vi "INV A - Current Sense Test_v2.vi"(8 "error in (no error)":errorcluster, 11 "Control Board VISA":refnum<visa-resource-name>) -> (0 "error out":errorcluster, 3 "Sense UVW":dbl[](array[numeric]))   [LabVIEW 2022 SP3]
uses:
  Serial Board Com/Board Select.ctl
  Serial Board Com/ADCSelector BB.ctl
  Serial Board Com/ADCSelector GB.ctl
panel:
  in  "Board Select":T1
  out "Sense W":dbl
  out "Sense V":dbl
  out "Sense U":dbl
  out "INVA_ISENSE_W":bool
  out "INVA_ISENSE_V":bool
  out "INVA_ISENSE_U":bool
  in  "Message IN":string
  out "Message OUT":string
  out "VISA OUT":refnum<visa-resource-name>
  out "Result (color)":u32(colorbox)
  out "Result (bool)":bool
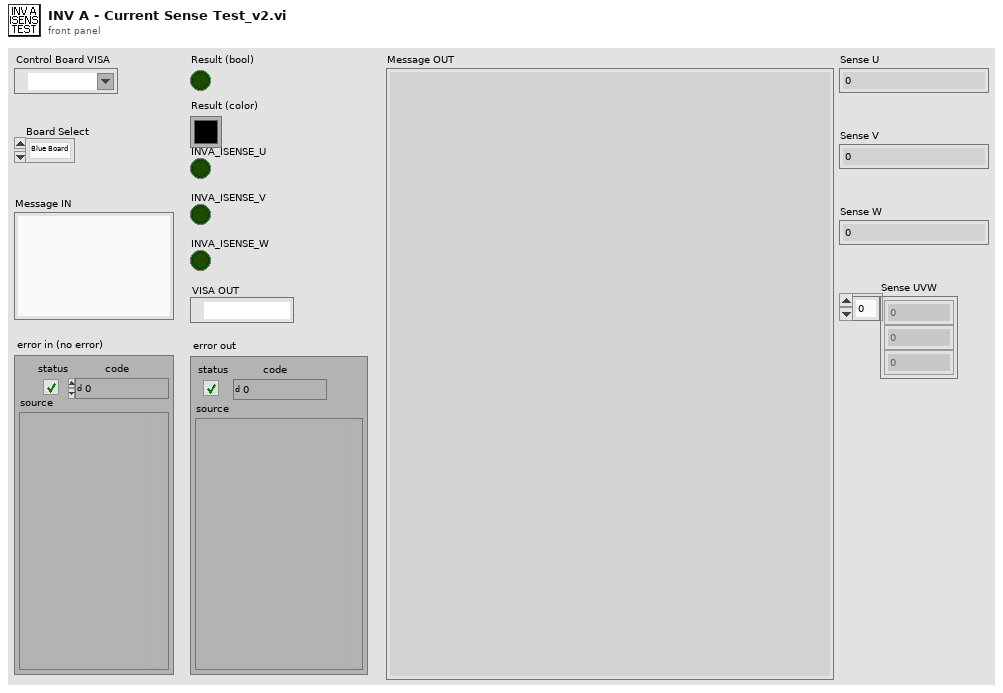
[diagram p1: front panel]
types:
  T1 = typedef "Board Select.ctl" = enum16{"Blue Board", "Green Board"}
  T2 = typedef "ADCSelector GB.ctl" = enum16{"INVA_ISENSE_U", "INVA_ISENSE_V", "INVA_ISENSE_W", "INVA_UDC", "INVA_TEMP", "HB_ISENSE", "AUX_ISENSE_U", "AUX_ISENSE_V", "AUX_ISENSE_W", "VLINE_AB", "VLINE_BC", "VLINE_CA", "REF_1P5V", "VSENSE_POS_24V", "VSENSE_POS_5V", "VSENSE_NEG_15V", "TEST_POINT", "INVB_ISENSE_U", "INVB_ISENSE_V", "INVB_ISENSE_W", "INVB_UDC", "INVB_TEMP", "HB_TEMP", "AUXA_TEMP", "AUXB_TEMP", "AUXC_TEMP", "VOUT_AB", "VOUT_BC", "VOUT_CA", "REF_2P5V", "VSENSE_POS_15V", "VSENSE_POS_3P3V", "NET_ANALYZER"}
  T3 = typedef "ADCSelector BB.ctl" = enum16{"INVA_ISENSE_U", "INVA_ISENSE_V", "INVA_ISENSE_W", "INVA_UDC", "INVA_TEMP", "HB_TEMP", "AUXB_TEMP", "VLINE_AB", "VLINE_BC", "VLINE_CA", "VSENSE_POS_24V", "VSENSE_POS_5V", "VSENSE_NEG_15V", "INVB_ISENSE_U", "INV_B_ISENSEV", "INVB_ISENSE_W", "INVB_UDC", "INVB_TEMP", "AUXA_TEMP", "AUXC_TEMP", "VOUT_AB", "VOUT_BC", "VOUT_CA", "VSENSE_POS_15V", "VSENSE_POS_3P3V", "TEST_POINT"}
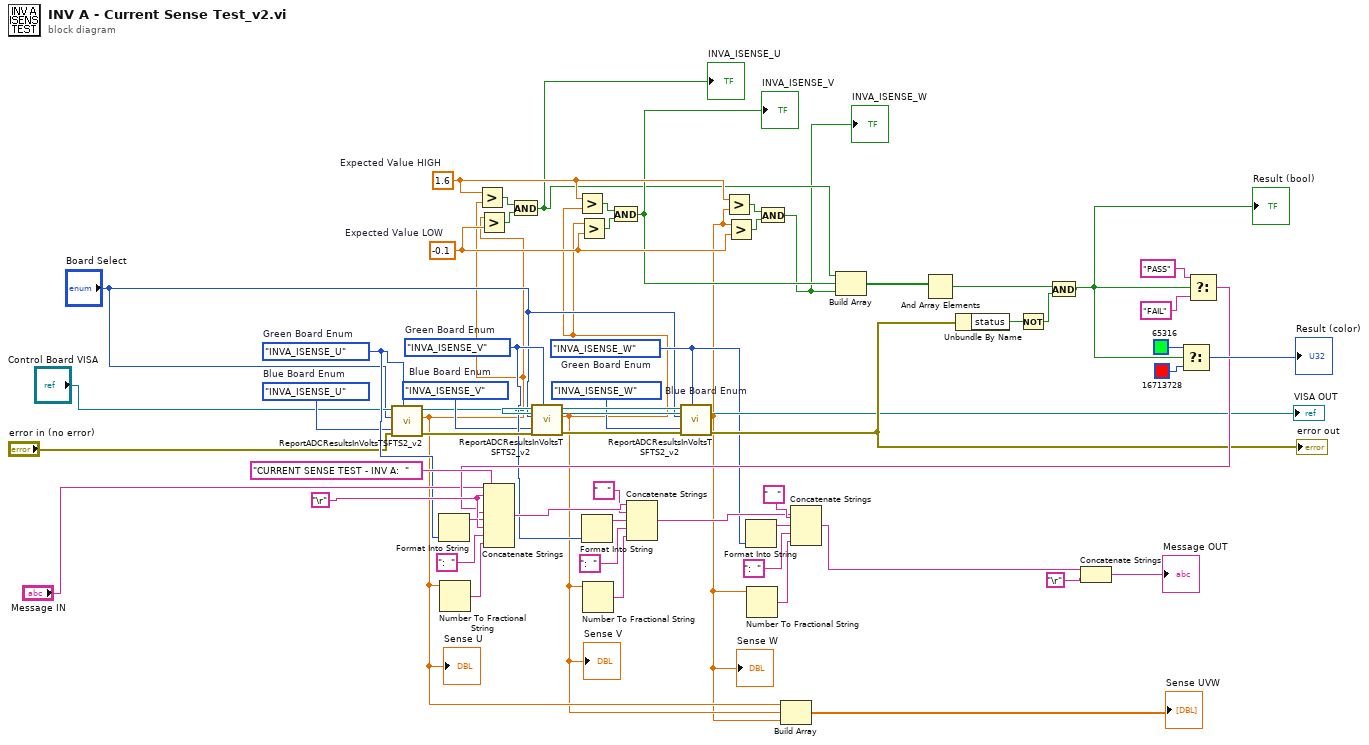
[diagram p0: block diagram]
diagram:
  w14 = ADCSelector_GB."INVA_ISENSE_W"  # Green Board Enum
  w15 = ADCSelector_GB."INVA_ISENSE_V"  # Green Board Enum
  w16 = ADCSelector_GB."INVA_ISENSE_U"  # Green Board Enum
  w21 = "\r"
  w36 = -0.1  # Expected Value LOW
  w35 = 1.6  # Expected Value HIGH
  w10 = ADCSelector_BB."INVA_ISENSE_W"  # Blue Board Enum
  w11 = ADCSelector_BB."INVA_ISENSE_V"  # Blue Board Enum
  w12 = ADCSelector_BB."INVA_ISENSE_U"  # Blue Board Enum
  n1 = call "ReportADCResultsInVoltsTSFTS2_v2.vi"("Blue Board Enum"=w12, "Green Board Enum"=w16, "error in (no error)"="error in (no error)", "Board Selector"="Board Select", "Control Board VISA"="Control Board VISA") -> ("error out"=w51:errorcluster, "Result"=w5:dbl, "Control Board VISA Out"=w7:refnum<visa-resource-name>)  [unwired: 3 in, 1 out]
  "Sense U" <- w5
  n2 = Format Into String(w16) -> (resulting string=w22:string)  [unwired: 3 in, 1 out]
  n3 = Number To Fractional String(number=w5) -> (F-format string=w24:string)  [unwired: 3 in]
  n4 = Greater?(x=w35, y=w5) -> (0:w42:bool)
  n5 = Greater?(x=w5, y=w36) -> (0:w41:bool)
  n6 = And(x=w42, y=w41) -> (x .and. y?=w33:bool)
  "INVA_ISENSE_U" <- w33
  n7 = call "ReportADCResultsInVoltsTSFTS2_v2.vi"("Blue Board Enum"=w11, "Green Board Enum"=w15, "error in (no error)"=w51, "Board Selector"="Board Select", "Control Board VISA"=w7) -> ("error out"=w50:errorcluster, "Result"=w4:dbl, "Control Board VISA Out"=w6:refnum<visa-resource-name>)  [unwired: 3 in, 1 out]
  "Sense V" <- w4
  n8 = Greater?(x=w35, y=w4) -> (0:w39:bool)
  n9 = Greater?(x=w4, y=w36) -> (0:w40:bool)
  n10 = Format Into String(w15) -> (resulting string=w47:string)  [unwired: 3 in, 1 out]
  n11 = Number To Fractional String(number=w4) -> (F-format string=w48:string)  [unwired: 3 in]
  n12 = And(x=w39, y=w40) -> (x .and. y?=w34:bool)
  "INVA_ISENSE_V" <- w34
  n13 = call "ReportADCResultsInVoltsTSFTS2_v2.vi"("Blue Board Enum"=w10, "Green Board Enum"=w14, "error in (no error)"=w50, "Board Selector"="Board Select", "Control Board VISA"=w6) -> ("error out"=w18:errorcluster, "Result"=w3:dbl, "Control Board VISA Out"=→"VISA OUT":refnum<visa-resource-name>)  [unwired: 3 in, 1 out]
  "error out" <- w18
  "Sense W" <- w3
  n14 = Greater?(x=w35, y=w3) -> (0:w38:bool)
  n15 = Greater?(x=w3, y=w36) -> (0:w37:bool)
  n16 = Format Into String(w14) -> (resulting string=w46:string)  [unwired: 3 in, 1 out]
  n17 = Number To Fractional String(number=w3) -> (F-format string=w45:string)  [unwired: 3 in]
  n18 = And(x=w38, y=w37) -> (x .and. y?=w32:bool)
  "INVA_ISENSE_W" <- w32
  n19 = Build Array(w5, w4, w3) -> (→"Sense UVW":dbl[])
  n20 = Build Array(w33, w34, w32) -> (w1:bool[])
  n21 = And Array Elements(Boolean array=w1) -> (logical AND=w54:bool)
  n22 = Unbundle By Name(w18) -> ("status"=w43:bool)
  n23 = Not(x=w43) -> (.not. x?=w53:bool)
  n24 = And(x=w54, y=w53) -> (x .and. y?=w55:bool)
  "Result (bool)" <- w55
  n25 = Select(t=u32 65316 ("Result (color)"), s=w55, f=u32 16713728 ("Result (color)")) -> (s? t:f=→"Result (color)":u32)
  n26 = Select(t="PASS", s=w55, f="FAIL") -> (s? t:f=w20:string)
  n27 = Concatenate Strings("Message IN", w21, "CURRENT SENSE TEST - INV A:  ", w20, w21, w22, ":  ", w24) -> (w31:string)
  n28 = Concatenate Strings(w31, "   ", w47, ":  ", w48) -> (w28:string)
  n29 = Concatenate Strings(w28, "   ", w46, ":  ", w45) -> (w27:string)
  n30 = Concatenate Strings(w27, "\r") -> (→"Message OUT":string)
